vi "get_xyz_position.vi"(8 "error in (no error)":errorcluster, 11 "Handle in":i64) -> (0 "error out":errorcluster, 1 "XYZ position (nm)":cluster{"x_pos":i32, "y_pos":i32, "z_pos":i32}, 2 "Return (<0 is error)":i32, 3 "Handle out":i64)   [LabVIEW 2016, in "OSB_uMp_library.lvlib"]
doc: "Returns uMp's position in nm. You must set the active manipulator using \"Select device.vi\" before calling this VI.\n\n\n!!!\nUsage warning\n!!!\nMay need to get recent information from the uMp before calling this VI. One way of doing this is to call the \"ping\" VI first."
uses:
  OSB_uMp_library.lvlib
  ump.dll
panel:
  # "By Stuart Box at OxSyBio Ltd, 2017\n\nThis software is provided WITHOUT ANY WARRANTY; without even the implied warranty of MERCHANTABILITY or FITNESS FOR A PARTICULAR PURPOSE.\n\ninfo@oxsybio.com\n\nOxSyBio Ltd, The Walbrook Building, 25 Walbrook, London, EC4N 8AF"
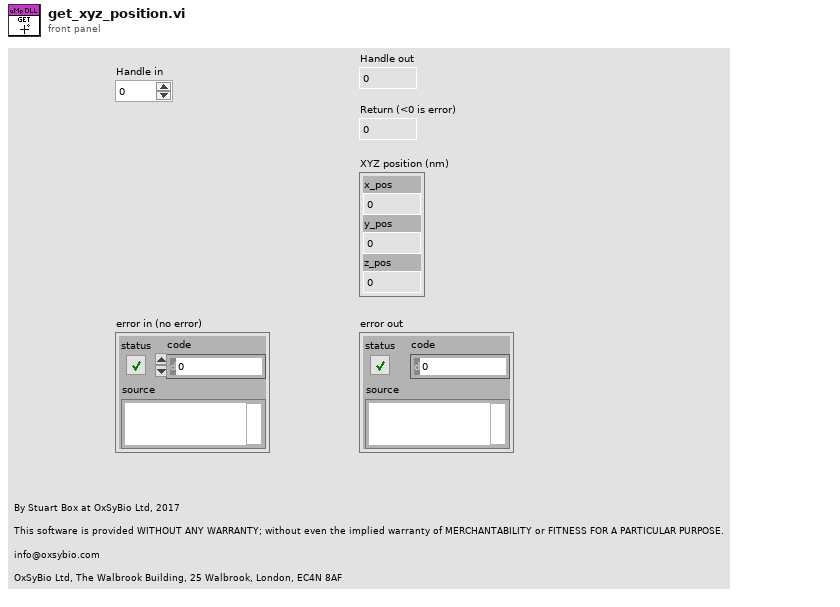
[diagram p1: front panel]
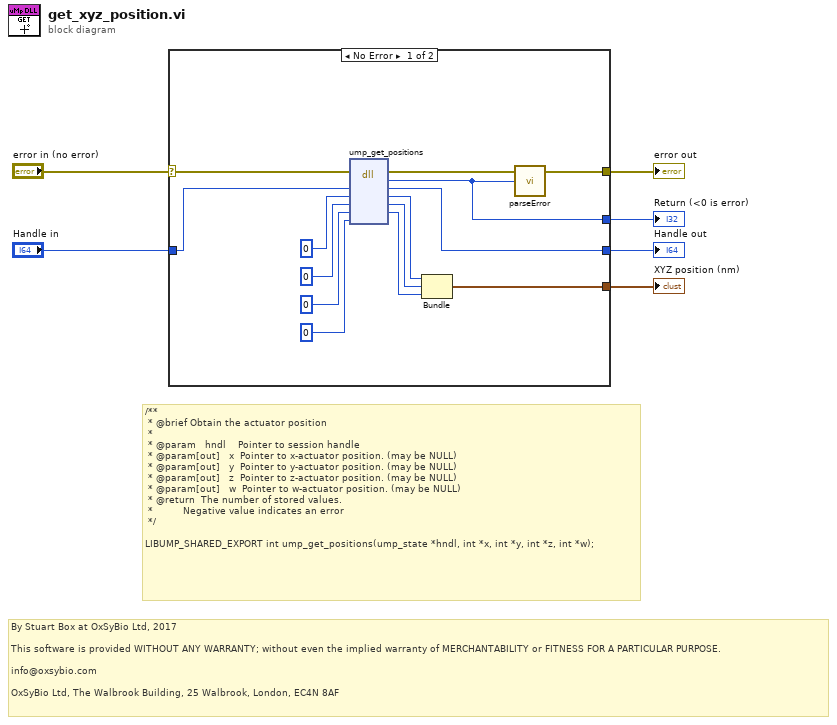
[diagram p0: block diagram]
diagram:
  # "By Stuart Box at OxSyBio Ltd, 2017\n\nThis software is provided WITHOUT ANY WARRANTY; without even the implied warranty of MERCHANTABILITY or FITNESS FOR A PARTICULAR PURPOSE.\n\ninfo@oxsybio.com\n\nOxSyBio Ltd, The Walbrook Building, 25 Walbrook, London, EC4N 8AF"
  # "/**\n * @brief Obtain the actuator position\n *\n * @param   hndl    Pointer to session handle\n * @param[out]   x  Pointer to x-actuator position. (may be NULL)\n * @param[out]   y  Pointer to y-actuator position. (may be NULL)\n * @param[out]   z  Pointer to z-actuator position. (may be NULL)\n * @param[out]   w  Pointer to w-actuator position. (may be NULL)\n * @return  The number of stored values.\n *          Negative value indicates an error\n */\n\nLIBUMP_SHARED_EXPORT int ump_get_positions(ump_state *hndl, int *x, int *y, int *z, int *w);"
  n1 = case shown="No Error" "error in (no error)" {
    selector: "error in (no error)" -> [w10 w22]
    tunnel: [w7 _] -> w6
    tunnel: [w8 w22] -> w5
    tunnel: [w20 _] -> w4
    tunnel: "Handle in" -> [w16 w21]
    tunnel: [w11 w21] -> w2
    frame No Error {
      n2 = dll-call lib="C:/Users/Stu/Desktop/OSB LabVIEW uMp/uMp_library/ump.dll" fn="ump_get_positions"(error in=w10, "handle"=w16, "x_pos"=0, "y_pos"=0, "z_pos"=0, "w_pos"=0) -> (error out=w9:errorcluster, "return"=w7:i32, "handle"=w11:i64, "x_pos"=w17:i32, "y_pos"=w18:i32, "z_pos"=w19:i32)  [unwired: 3 in, 1 out]
      n3 = Bundle("x_pos"=w17, "y_pos"=w18, "z_pos"=w19) -> (w20:cluster{"x_pos":i32, "y_pos":i32, "z_pos":i32})  [unwired: 1 in]
      n4 = call "parseError.vi"("Error In"=w9, "ump dll return value (<0 is error)"=w7) -> ("Error Out"=w8:errorcluster)  [unwired: 24 in, 1 out]
    }
    frame Error {
    }
  }
  "Return (<0 is error)" <- w6
  "error out" <- w5
  "XYZ position (nm)" <- w4
  "Handle out" <- w2
